vi "Init FIFOs (STM Multi-Client).vi"(8 "error in (no error)":errorcluster) -> (0 "error out":errorcluster, 3 "FIFOs out":T1)   [LabVIEW 2010]
uses:
  FIFOs (STM Multi-Client).ctl
panel:
  in  "FIFOs dummy":T1
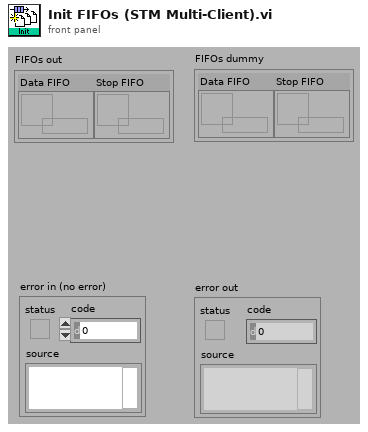
[diagram p1: front panel]
types:
  T1 = typedef "FIFOs (STM Multi-Client).ctl" = cluster{"Data FIFO":refnum<queue>, "Stop FIFO":refnum<queue>}
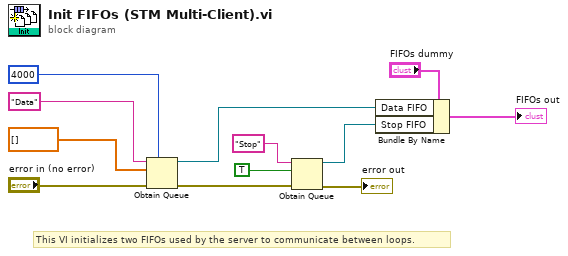
[diagram p0: block diagram]
diagram:
  # "This VI initializes two FIFOs used by the server to communicate between loops."
  n1 = Obtain Queue(max queue size (-1, unlimited)=4000 ("elements in array (1)"), name (unnamed)="Data", element data type=dbl[] [], error in (no error)="error in (no error)") -> (queue out=w8:refnum<queue>, error out=w11:errorcluster)  [unwired: 1 in, 1 out]
  n2 = Obtain Queue(name (unnamed)="Stop", element data type=TRUE, error in (no error)=w11) -> (queue out=w9:refnum<queue>, error out=→"error out":errorcluster)  [unwired: 2 in, 1 out]
  n3 = Bundle By Name(cluster="FIFOs dummy", "Data FIFO"=w8, "Stop FIFO"=w9) -> (→"FIFOs out":T1)
